vi "test_libssh2_channel_read.vi"() -> ()   [LabVIEW 2017, in "integration_tests.lvlib"]
uses:
  integration_tests.lvlib
  libssh2/libssh2_channel_open_ex.vi
  libssh2/libssh2_channel_process_startup.vi
  libssh2/libssh2_channel_read_ex.vi
  support/support.lvlib
  libssh2/libssh2.lvlib
  <vilib>/PNR/Transparent Assertions/Transparent Assertions/Transparent Assertions.lvlib
panel:
  out "error out":errorcluster
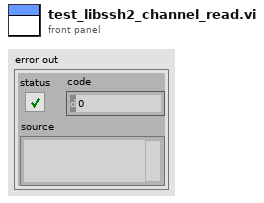
[diagram p1: front panel]
types:
  T1 = typedef "libssh2.lvlib/Session Refnum.ctl" = refnum<k1>
  T2 = typedef "libssh2.lvlib/Channel Refnum.ctl" = refnum<k1>
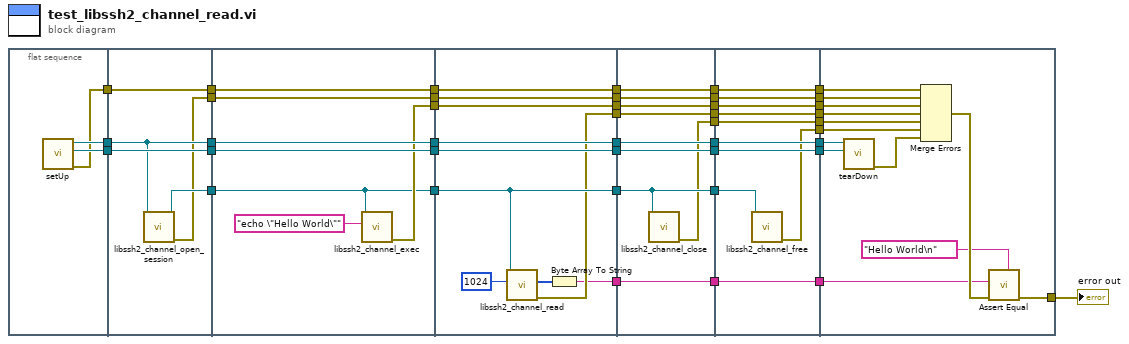
[diagram p0: block diagram]
diagram:
  n1 = flat-sequence {
    tunnel: [w44] -> w41
    tunnel: [w43] -> w40
    tunnel: [w42] -> w39
    tunnel: w41 -> [w48]
    tunnel: w40 -> [w49]
    tunnel: [w48] -> w24
    tunnel: [w49] -> w23
    tunnel: [w47] -> w22
    tunnel: w39 -> [w46]
    tunnel: [w46] -> w21
    tunnel: [w45] -> w20
    tunnel: w24 -> [w56]
    tunnel: [w56] -> w17
    tunnel: w23 -> [w55]
    tunnel: [w55] -> w15
    tunnel: w22 -> [w50]
    tunnel: [w50] -> w13
    tunnel: w21 -> [w54]
    tunnel: [w54] -> w11
    tunnel: w20 -> [w53]
    tunnel: [w53] -> w9
    tunnel: [w51] -> w7
    tunnel: w17 -> [w66]
    tunnel: [w66] -> w16
    tunnel: w15 -> [w65]
    tunnel: [w65] -> w14
    tunnel: w13 -> [w60]
    tunnel: [w60] -> w12
    tunnel: w11 -> [w64]
    tunnel: [w64] -> w10
    tunnel: w9 -> [w63]
    tunnel: [w63] -> w8
    tunnel: w7 -> [w62]
    tunnel: [w62] -> w6
    tunnel: [w59] -> w5
    tunnel: [w57] -> w2
    tunnel: w16 -> [w75]
    tunnel: w14 -> [w74]
    tunnel: w12 -> [w73]
    tunnel: [w75] -> w38
    tunnel: [w74] -> w37
    tunnel: [w67] -> w36
    tunnel: [w73] -> w35
    tunnel: [w72] -> w34
    tunnel: w10 -> [w71]
    tunnel: [w71] -> w33
    tunnel: w8 -> [w70]
    tunnel: [w70] -> w26
    tunnel: w6 -> [w69]
    tunnel: [w69] -> w19
    tunnel: w5 -> [w68]
    tunnel: [w68] -> w4
    tunnel: w2 -> [w67]
    tunnel: w38 -> [w85]
    tunnel: w37 -> [w84]
    tunnel: w36 -> [w83]
    tunnel: w35 -> [w82]
    tunnel: [w85] -> w32
    tunnel: [w84] -> w31
    tunnel: [w83] -> w30
    tunnel: [w81] -> w29
    tunnel: w34 -> [w80]
    tunnel: [w80] -> w28
    tunnel: w33 -> [w79]
    tunnel: [w79] -> w27
    tunnel: w26 -> [w78]
    tunnel: [w78] -> w25
    tunnel: w19 -> [w77]
    tunnel: [w77] -> w18
    tunnel: w4 -> [w76]
    tunnel: [w76] -> w3
    tunnel: w32 -> [w98]
    tunnel: w31 -> [w97]
    tunnel: w30 -> [w87]
    tunnel: [w96] -> w1
    tunnel: w29 -> [w94]
    tunnel: w28 -> [w93]
    tunnel: w27 -> [w92]
    tunnel: w25 -> [w90]
    tunnel: w18 -> [w89]
    tunnel: w3 -> [w88]
    frame #0 {
      n2 = call "setUp.vi"() -> ("error out"=w42:errorcluster, "connection ID"=w43:refnum<k5>, "session"=w44:T1)  [unwired: 9 in]
    }
    frame #1 {
      n3 = call "libssh2_channel_open_session.vi"("session"=w48) -> ("error out"=w45:errorcluster, "channel"=w47:T2)  [unwired: 9 in]
    }
    frame #2 {
      n4 = call "libssh2_channel_exec.vi"("command"="echo \"Hello World\"", "channel"=w50) -> ("error out"=w51:errorcluster)  [unwired: 9 in]
    }
    frame #3 {
      n5 = call "libssh2_channel_read.vi"("buffer length"=1024, "channel"=w60) -> ("error out"=w59:errorcluster, "buffer"=w58:u8[])  [unwired: 8 in]
      n6 = Byte Array To String(unsigned byte array=w58) -> (string=w57:string)
    }
    frame #4 {
      n7 = call "libssh2_channel_close.vi"("channel"=w73) -> ("error out"=w72:errorcluster)  [unwired: 10 in]
    }
    frame #5 {
      n8 = call "libssh2_channel_free.vi"("channel"=w82) -> ("error out"=w81:errorcluster)  [unwired: 10 in]
    }
    frame #6 {
      n9 = call "tearDown.vi"("connection ID"=w97, "session"=w98) -> ("error out"=w95:errorcluster)  [unwired: 9 in]
      n10 = Merge Errors(w92, w90, w89, w88, w93, w94, w95) -> (w91:errorcluster)
      n11 = call <vilib>:"Assert Equal.vi"("Expected"="Hello World\n", "error in (no error)"=w91, "Actual"=w87) -> ("error out"=w96:errorcluster)  [unwired: 8 in]
    }
  }
  "error out" <- w1
